vi "Sub_Build_Variable_Header_Publish.vi"(8 "error in (no error)":errorcluster, 9 "Message ID":u16=1 format="%x", 10 "Topic Name":string="Topic", 11 "QoS":T1) -> (0 "error out":errorcluster, 2 "Variable Header":u8[](array[numeric]) format="%x")   [LabVIEW 2018, in "MQTT_Functions.lvlib"]
uses:
  MQTT_Functions.lvlib
  Controls/QoS.ctl
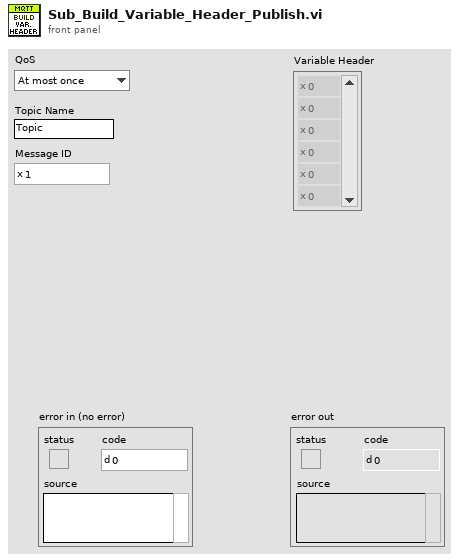
[diagram p1: front panel]
types:
  T1 = typedef "MQTT_Functions.lvlib/QoS.ctl" = enum8{"At most once", "At least once", "Exactly once", "Reserved"}
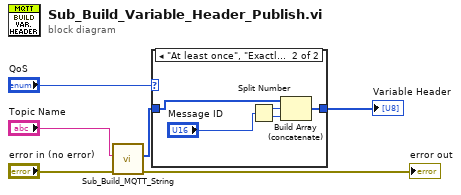
[diagram p0: block diagram]
diagram:
  n1 = call "Sub_Build_MQTT_String.vi"("error in (no error)"="error in (no error)", "String to be encoded"="Topic Name") -> ("error out"=→"error out":errorcluster, "UTF8 Byte Array"=w2:u8[])  [unwired: 8 in]
  n2 = case shown="\"At least once\", \"Exactly once\"" "QoS" {
    tunnel: w2 -> [w7 w12]
    tunnel: [w7 w11] -> w1
    frame "At most once", Default {
      # "no message id"
    }
    frame "At least once", "Exactly once" {
      n3 = Split Number(x="Message ID") -> (hi(x)=w9:u8, lo(x)=w8:u8)
      n4 = Build Array (concatenate)(w12, w9, w8) -> (w11:u8[])
    }
  }
  "Variable Header" <- w1
